vi "Cartesian To Polar.vi"(8 "Joystick y axis input":dbl, 10 "Joystick x axis input":dbl) -> (0 "Theta (deg)":dbl, 2 "Magnitude":dbl)   [LabVIEW 2018]
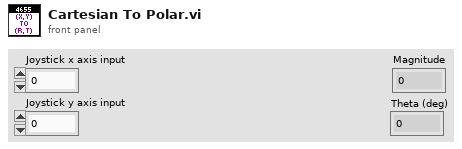
[diagram p1: front panel]
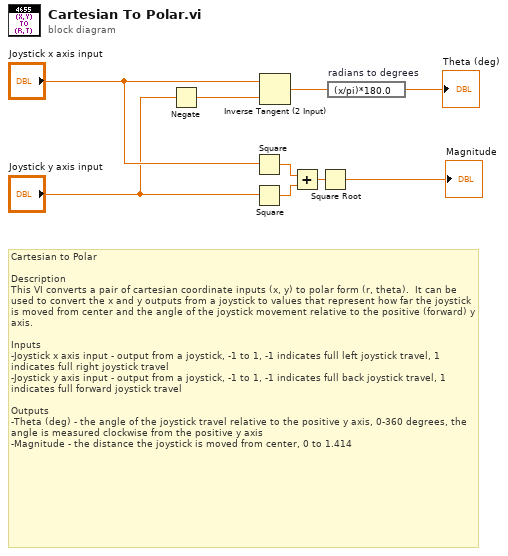
[diagram p0: block diagram]
diagram:
  # "Cartesian to Polar\n\nDescription\nThis VI converts a pair of cartesian coordinate inputs (x, y) to polar form (r, theta).  It can be used to convert the x and y outputs from a joystick to values that represent how far the joystick is moved from center and the angle of the joystick movement relative to the positive (forward) y axis.\n\nInputs\n-Joystick x axis input - output from a joystick, -1 to 1, -1 indicates full left joystick travel, 1 indicates full right joystick travel\n-Joystick y axis input - output from a joystick, -1 to 1, -1 indicates full back joystick travel, 1 indicates full forward joystick travel\n\nOutputs\n-Theta (deg) - the angle of the joystick travel relative to the positive y axis, 0-360 degrees, the angle is measured clockwise from the positive y axis\n-Magnitude - the distance the joystick is moved from center, 0 to 1.414"
  n1 = Negate(x="Joystick y axis input") -> (-x=w3:dbl)
  n2 = Square(x="Joystick x axis input") -> (x^2=w8:dbl)
  n3 = Square(x="Joystick y axis input") -> (x^2=w7:dbl)
  n4 = Inverse Tangent (2 Input)(1:w3, 2:"Joystick x axis input") -> (0:w9:dbl)
  n5 = Add(x=w8, y=w7) -> (x+y=w6:dbl)
  n6 = Square Root(x=w6) -> (sqrt(x)=→"Magnitude":dbl)
  n7 = expression code="(x/pi)*180.0" "radians to degrees"(w9) -> (→"Theta (deg)":dbl)
